vi "LESO_write.vi"(8 "error in":errorcluster, 9 "Bytes To Write":u32, 10 "Buffer":u8[](array[numeric]), 11 "Handle in":u32) -> (0 "error out":errorcluster, 1 "Bytes Written":u32, 2 "FT_Status":u32(ring) items=["FT_OK", "FT_INVALID_HANDLE", "FT_DEVICE_NOT_FOUND", "FT_DEVICE_NOT_OPENED", "FT_IO_ERROR", "FT_INSUFFICIENT_RESOURCES", "FT_INVALID_PARAMETER", "FT_INVALID_BAUD_RATE", "FT_DEVICE_NOT_OPENED_FOR_ERASE", "FT_DEVICE_NOT_OPENED_FOR_WRITE", "FT_FAILED_TO_WRITE_DEVICE", "FT_EEPROM_READ_FAILED", "FT_EEPROM_WRITE_FAILED", "FT_EEPROM_ERASE_FAILED", "FT_EEPROM_NOT_PRESENT", "FT_EEPROM_NOT_PROGRAMMED", "FT_INVALID_ARGS", "FT_NOT_SUPPORTED", "FT_OTHER_ERROR"], 3 "Handle out":u32)   [LabVIEW 2012]
doc: "Передает массив данных устройству."
uses:
  FTD2XX.dll
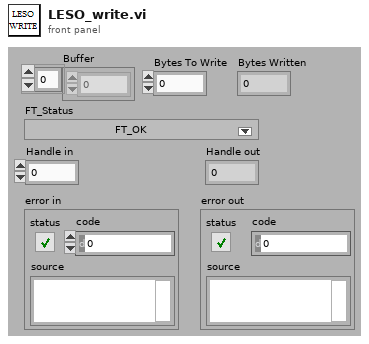
[diagram p1: front panel]
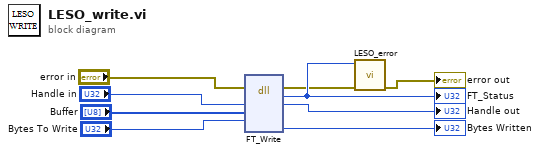
[diagram p0: block diagram]
diagram:
  n1 = dll-call lib="FTD2XX.dll" fn="FT_Write"(error in="error in", "Handle"="Handle in", "Buffer"="Buffer", "BytesToWrite"="Bytes To Write") -> (error out=w5:errorcluster, "FT_Status"=w6:u32, "Handle"=→"Handle out":u32, "BytesWritten"=→"Bytes Written":u32)  [unwired: 5 in, 1 out]
  "FT_Status" <- w6
  n2 = call "LESO_error.vi"("error in"=w5, "FT_Status"=w6) -> ("error out"=→"error out":errorcluster)  [unwired: 9 in]
